vi "WriteOdorFileheader.vi"(11 "Byte Stream File in":refnum<file>) -> (3 "Byte Stream File out":refnum<file>)   [LabVIEW 2019]
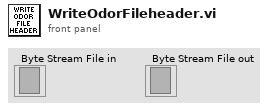
[diagram p1: front panel]
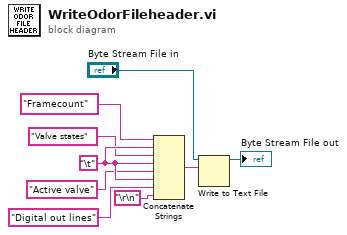
[diagram p0: block diagram]
diagram:
  w5 = "\t"
  n1 = Concatenate Strings("Framecount" ("text"), w5, "Valve states" ("string"), w5, "Active valve" ("string"), w5, "Digital out lines" ("string"), "\r\n") -> (w6:string)
  n2 = Write to Text File(file (use dialog)="Byte Stream File in", text=w6) -> (refnum out=→"Byte Stream File out":refnum<file>)  [unwired: 2 in, 2 out]
